vi "Get_Devices.vi"(8 "error in (no error)":errorcluster) -> (0 "error out":errorcluster, 2 "devices":T1(array[cluster]))   [LabVIEW 2019, in "Kinova MICO² USB.lvlib"]
uses:
  <vilib>/Utility/error.llb/Error Cluster From Error Code.vi
  <vilib>/ErrorRing/Error Ring.xnode
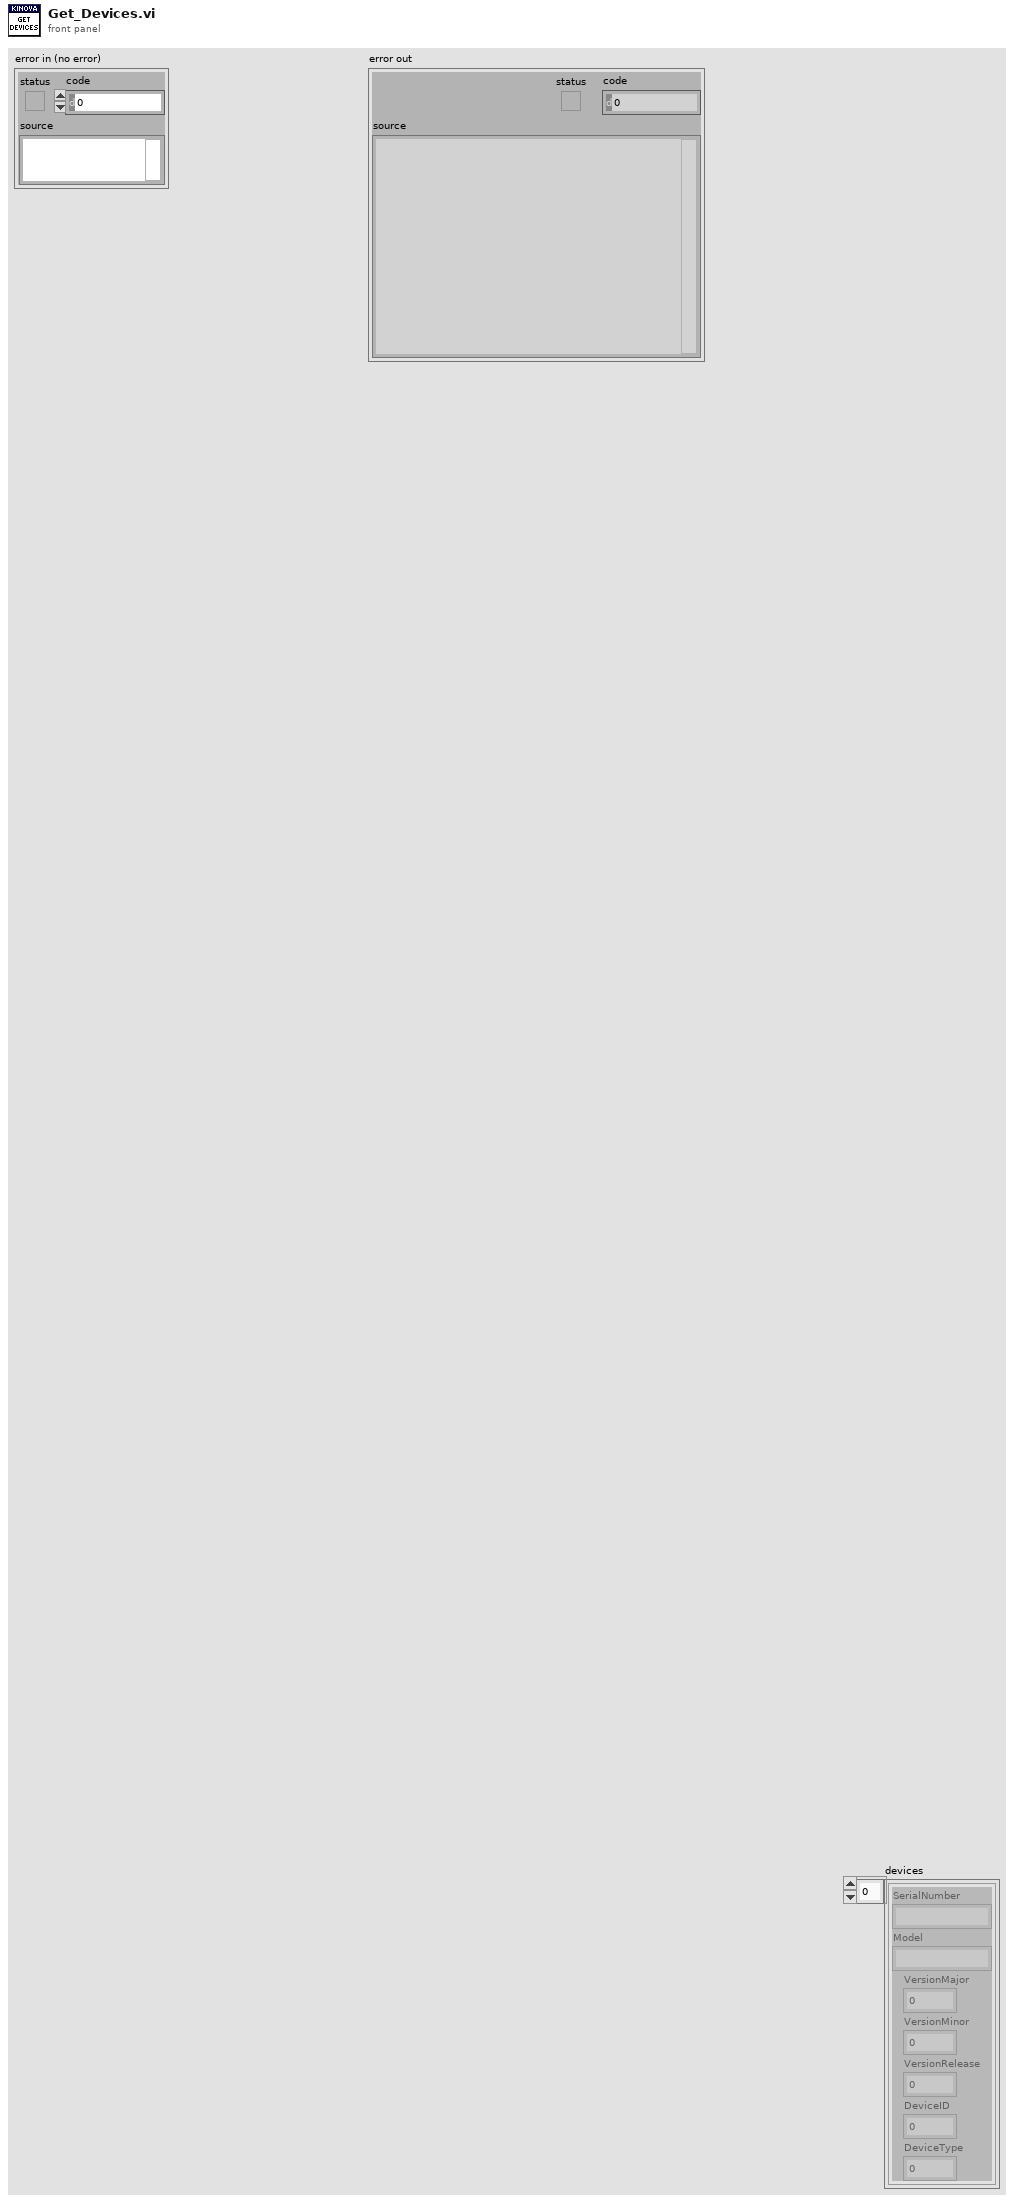
[diagram p1: front panel]
types:
  T1 = cluster{"SerialNumber":string, "Model":string, "VersionMajor":i32, "VersionMinor":i32, "VersionRelease":i32, "DeviceID":i32, "DeviceType":i32}[]
  T2 = cluster{"SerialNumber":string, "Model":string, "VersionMajor":i32, "VersionMinor":i32, "VersionRelease":i32, "DeviceID":i32, "DeviceType":i32}
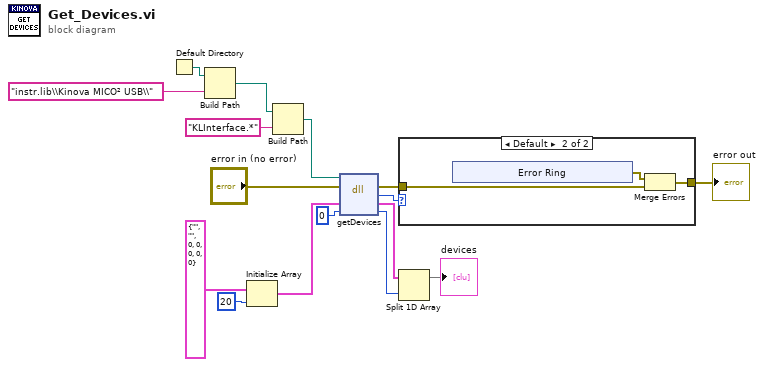
[diagram p0: block diagram]
diagram:
  n1 = Default Directory() -> (w3:path)
  n2 = Build Path(base path=w3, name or relative path="instr.lib\\Kinova MICO² USB\\") -> (appended path=w1:path)
  n3 = Initialize Array(T2 {"SerialNumber"="", "Model"="", "VersionMajor"=0, "VersionMinor"=0, "VersionRelease"=0, "DeviceID"=0, "DeviceType"=0} ("Kinova Device"), 20 ("dimension size")) -> (w10:T1)
  n4 = Build Path(base path=w1, name or relative path="KLInterface.*") -> (appended path=w4:path)
  n5 = dll-call lib="C:/Users/mcjssdcc/source/repos/Kinova Labview Interface/Debug/KLInterface.dll" fn="getDevices"(path in=w4, error in="error in (no error)", "devices"=w10, "devicecount"=0) -> (error out=w14:errorcluster, "return type"=w12:i32, "devices"=w7:T1, "devicecount"=w8:i32)  [unwired: 1 in, 1 out]
  n6 = case shown="Default" w12 {
    tunnel: [w17 w19] -> w13
    tunnel: w14 -> [w17 w18]
    frame 1 {
    }
    frame Default {
      n7 = xnode "Error Ring"() -> ("error out"=w20:errorcluster)
      n8 = Merge Errors(w20, w18) -> (w19:errorcluster)
    }
  }
  "error out" <- w13
  n9 = Split 1D Array(array=w7, index=w8) -> (first subarray=→"devices":T1)  [unwired: 1 out]
